vi "Read Data.vi"(8 "error in (no error)":errorcluster, 11 "Temp01 in":refnum<class "TELLC_Temp01.lvclass">) -> (0 "error out":errorcluster, 2 "Temp01ReadData":T1, 3 "Temp01 out":refnum<class "TELLC_Temp01.lvclass">)   [LabVIEW 2017, in "TELLC_Temp01.lvclass"]
doc: "Developed by Kevin Thompson\nkevin@thompsonengineering.net\n\nCopyright 2018\nThompson Engineering, LLC"
uses:
  TELLC_Temp01.lvclass
  DataTypes/Read Data--cluster.ctl
  TELLC_Temp01.lvclass/TELLC_Temp01.ctl
  Accessors/Set ReadData.vi
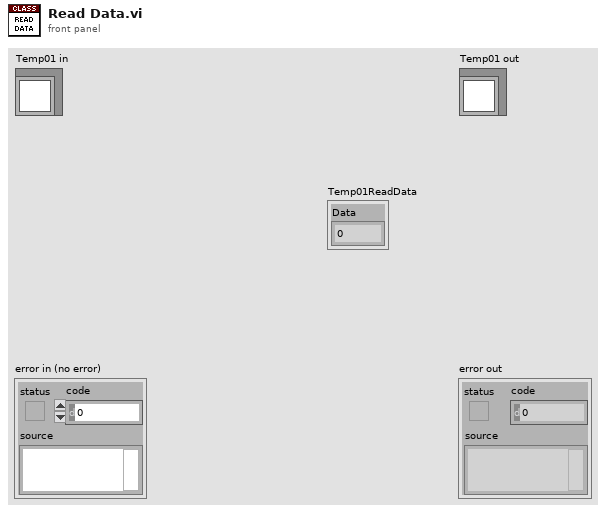
[diagram p1: front panel]
types:
  T1 = typedef "TELLC_Temp01.lvclass/Read Data--cluster.ctl" = cluster{"Data":dbl}
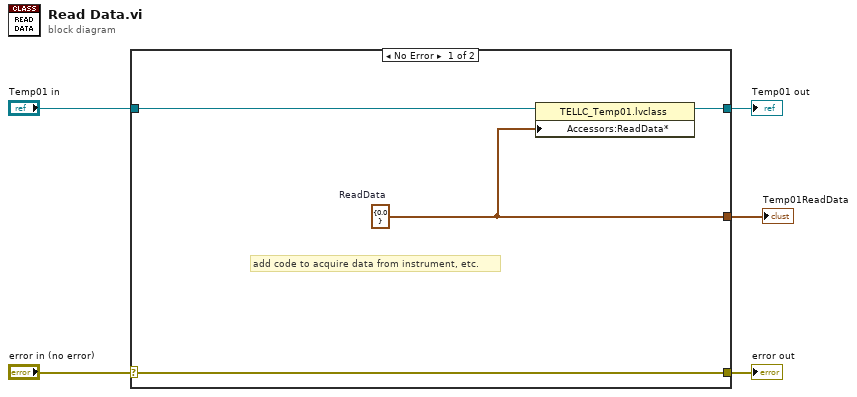
[diagram p0: block diagram]
diagram:
  n1 = case shown="No Error" "error in (no error)" {
    selector: "error in (no error)" -> [w9 w11]
    tunnel: [w9 w11] -> w4
    tunnel: [w7 w10] -> w2
    tunnel: "Temp01 in" -> [w8 w10]
    tunnel: [w6 _] -> w1
    frame No Error {
      w6 = T1 {"Data"=0.0}  # ReadData
      # "add code to acquire data from instrument, etc."
      n2 = property class="TELLC_Temp01.lvclass"(reference=w8, "Accessors:ReadData*"=w6) -> (reference out=w7:refnum<class "TELLC_Temp01.lvclass">)  [unwired: 1 in, 1 out]
    }
    frame Error {
    }
  }
  "error out" <- w4
  "Temp01 out" <- w2
  "Temp01ReadData" <- w1
